vi "semaphore.vi"() -> ()   [LabVIEW 2019]
panel:
  out ".not. x? 4":bool
  out ".not. x? 3":bool
  out ".not. x? 2":bool
  out ".not. x?":bool
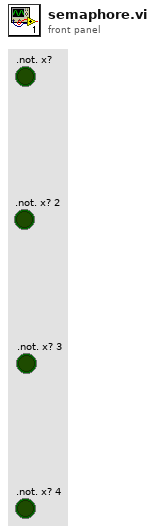
[diagram p1: front panel]
types:
  T1 = typedef "Semaphore RefNum" = refnum<k1>
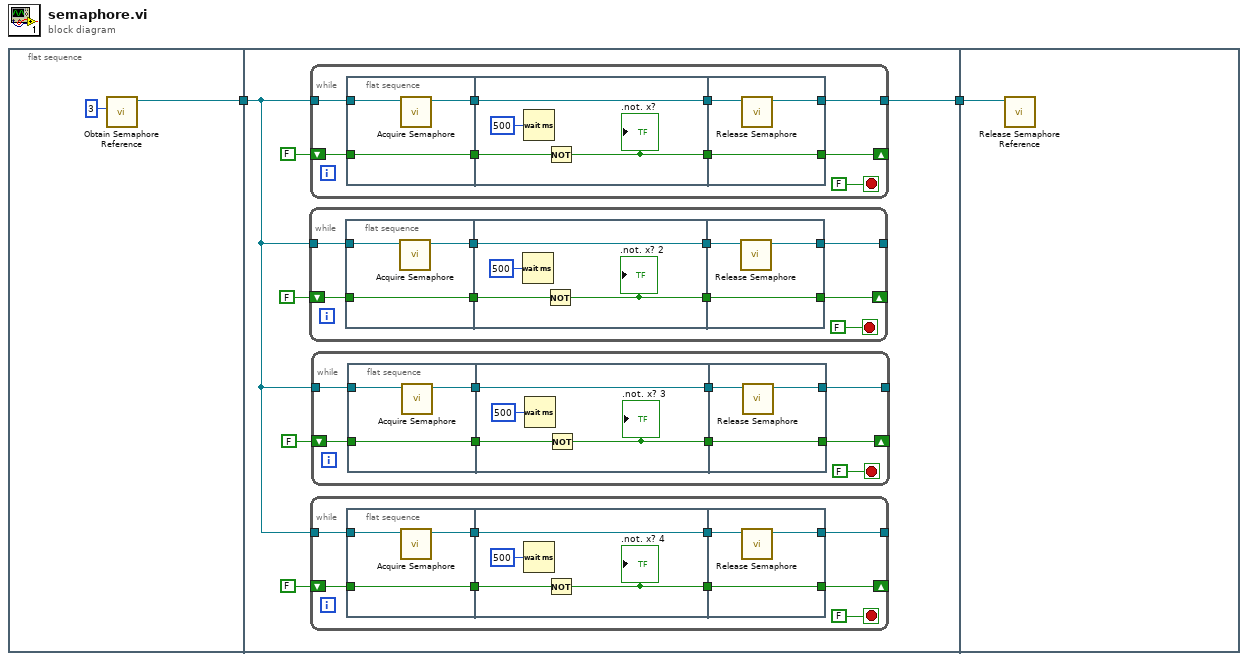
[diagram p0: block diagram]
diagram:
  n1 = flat-sequence {
    tunnel: [w3] -> w2
    tunnel: w2 -> [w5]
    tunnel: [w10] -> w1
    tunnel: w1 -> [w87]
    frame #0 {
      n2 = call <vilib>:"Obtain Semaphore Reference.vi"("size (1)"=3) -> ("semaphore"=w3:T1)  [unwired: 4 in, 2 out]
    }
    frame #1 {
      n3 = while {
        tunnel: w5 -> [w56]
        tunnel: [w53] -> _
        shift-right: [w49] -> _
        shift-left: FALSE -> [w52]
        stop <- FALSE stop-if-true
        n4 = flat-sequence {
          tunnel: w56 -> [w60]
          tunnel: [w59] -> w55
          tunnel: w52 -> [w58]
          tunnel: [w58] -> w51
          tunnel: w55 -> [w63]
          tunnel: [w63] -> w54
          tunnel: w51 -> [w62]
          tunnel: [w61] -> w50
          tunnel: w54 -> [w67]
          tunnel: [w66] -> w53
          tunnel: w50 -> [w65]
          tunnel: [w65] -> w49
          frame #0 {
            n5 = call <vilib>:"Acquire Semaphore.vi"("semaphore"=w60) -> ("semaphore out"=w59:T1)  [unwired: 4 in, 2 out]
          }
          frame #1 {
            n6 = Wait (ms)(milliseconds to wait=u32 500) -> ()  [unwired: 1 out]
            n7 = Not(x=w62) -> (.not. x?=w61:bool)
            ".not. x? 2" <- w61
          }
          frame #2 {
            n8 = call <vilib>:"Release Semaphore.vi"("semaphore"=w67) -> ("semaphore out"=w66:T1)  [unwired: 5 in, 1 out]
          }
        }
      }
      n9 = while {
        tunnel: w5 -> [w75]
        tunnel: [w72] -> w10
        shift-right: [w68] -> _
        shift-left: FALSE -> [w71]
        stop <- FALSE stop-if-true
        n10 = flat-sequence {
          tunnel: w75 -> [w79]
          tunnel: [w78] -> w74
          tunnel: w71 -> [w77]
          tunnel: [w77] -> w70
          tunnel: w74 -> [w82]
          tunnel: [w82] -> w73
          tunnel: w70 -> [w81]
          tunnel: [w80] -> w69
          tunnel: w73 -> [w86]
          tunnel: [w85] -> w72
          tunnel: w69 -> [w84]
          tunnel: [w84] -> w68
          frame #0 {
            n11 = call <vilib>:"Acquire Semaphore.vi"("semaphore"=w79) -> ("semaphore out"=w78:T1)  [unwired: 4 in, 2 out]
          }
          frame #1 {
            n12 = Wait (ms)(milliseconds to wait=u32 500) -> ()  [unwired: 1 out]
            n13 = Not(x=w81) -> (.not. x?=w80:bool)
            ".not. x?" <- w80
          }
          frame #2 {
            n14 = call <vilib>:"Release Semaphore.vi"("semaphore"=w86) -> ("semaphore out"=w85:T1)  [unwired: 5 in, 1 out]
          }
        }
      }
      n15 = while {
        tunnel: w5 -> [w18]
        tunnel: [w15] -> _
        shift-right: [w11] -> _
        shift-left: FALSE -> [w14]
        stop <- FALSE stop-if-true
        n16 = flat-sequence {
          tunnel: w18 -> [w22]
          tunnel: [w21] -> w17
          tunnel: w14 -> [w20]
          tunnel: [w20] -> w13
          tunnel: w17 -> [w25]
          tunnel: [w25] -> w16
          tunnel: w13 -> [w24]
          tunnel: [w23] -> w12
          tunnel: w16 -> [w29]
          tunnel: [w28] -> w15
          tunnel: w12 -> [w27]
          tunnel: [w27] -> w11
          frame #0 {
            n17 = call <vilib>:"Acquire Semaphore.vi"("semaphore"=w22) -> ("semaphore out"=w21:T1)  [unwired: 4 in, 2 out]
          }
          frame #1 {
            n18 = Wait (ms)(milliseconds to wait=u32 500) -> ()  [unwired: 1 out]
            n19 = Not(x=w24) -> (.not. x?=w23:bool)
            ".not. x? 4" <- w23
          }
          frame #2 {
            n20 = call <vilib>:"Release Semaphore.vi"("semaphore"=w29) -> ("semaphore out"=w28:T1)  [unwired: 5 in, 1 out]
          }
        }
      }
      n21 = while {
        tunnel: w5 -> [w37]
        tunnel: [w34] -> _
        shift-right: [w30] -> _
        shift-left: FALSE -> [w33]
        stop <- FALSE stop-if-true
        n22 = flat-sequence {
          tunnel: w37 -> [w41]
          tunnel: [w40] -> w36
          tunnel: w33 -> [w39]
          tunnel: [w39] -> w32
          tunnel: w36 -> [w44]
          tunnel: [w44] -> w35
          tunnel: w32 -> [w43]
          tunnel: [w42] -> w31
          tunnel: w35 -> [w48]
          tunnel: [w47] -> w34
          tunnel: w31 -> [w46]
          tunnel: [w46] -> w30
          frame #0 {
            n23 = call <vilib>:"Acquire Semaphore.vi"("semaphore"=w41) -> ("semaphore out"=w40:T1)  [unwired: 4 in, 2 out]
          }
          frame #1 {
            n24 = Wait (ms)(milliseconds to wait=u32 500) -> ()  [unwired: 1 out]
            n25 = Not(x=w43) -> (.not. x?=w42:bool)
            ".not. x? 3" <- w42
          }
          frame #2 {
            n26 = call <vilib>:"Release Semaphore.vi"("semaphore"=w48) -> ("semaphore out"=w47:T1)  [unwired: 5 in, 1 out]
          }
        }
      }
    }
    frame #2 {
      n27 = call <vilib>:"Release Semaphore Reference.vi"("semaphore"=w87) -> ()  [unwired: 9 in, 2 out]
    }
  }
